vi "Select Device.vi"() -> ()   [LabVIEW 2020]
panel:
  in  "Singing Helmet":bool
  in  "Redirect":bool
  in  "Collection":bool
  in  "Incomplete":bool
  # "Pick an Device"
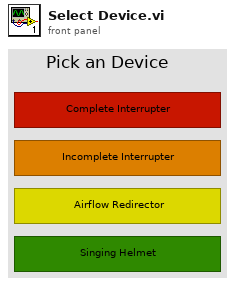
[diagram p1: front panel]
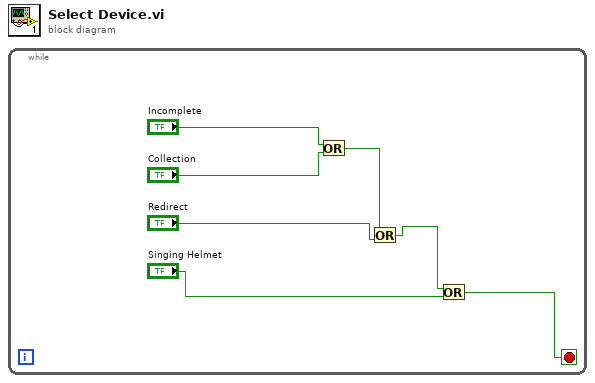
[diagram p0: block diagram]
diagram:
  n1 = while {
    stop <- w1 stop-if-true
    n2 = Or(x="Incomplete", y="Collection") -> (x .or. y?=w5:bool)
    n3 = Or(x=w5, y="Redirect") -> (x .or. y?=w3:bool)
    n4 = Or(x=w3, y="Singing Helmet") -> (x .or. y?=w1:bool)
  }
